vi "main_1 displacement detection.vi"() -> ()   [LabVIEW 2024]
doc: "This example shows how to configure multiple channels and acquire waveforms from multiple channels."
uses:
  RIGOL DS5000 7000 8000 Series/Public/Data/Read Waveform (Multiple).vi
  <vilib>/measure/mamon.llb/Waveform Peak Detection for 1 Chan.vi
  <vilib>/express/express analysis/Spectral/Block/exnSpectralBlock spectral measurements peak poly.vi
  <vilib>/express/express analysis/Spectral/Block/exnSpectralBlock spectral measurements peak WFM.vi
  <vilib>/Utility/file.llb/Write Delimited Spreadsheet (string).vi
  <vilib>/express/express analysis/Spectral/XNode/ExpressSpectralMeasurementsBlockNode.xnode
  RIGOL DS5000 7000 8000 Series/RIGOL DS5000 7000 8000 Series.lvlib
  <vilib>/measure/NI_MAPro.lvlib
panel:
  in  "Reset":bool
  in  "Negative direction":bool
  out "位移":dbl(graph)
  out "字符串":string
  in  "确定按钮":bool
  out "布尔 2":bool
  in  "Threshold":dbl=0.15
  in  "Save":bool
  out "Frequency":dbl
  in  "Time":dbl=20.0
  out "下拉列表":u16(ring)
  out "Count":dbl
  out "0, 1":i16
  out "子数组":dbl[](array[numeric])
  out "大小":i32
  out "# found":i32 caption="Count"
  in  "记时长度":dbl format="%#_13g"
  in  "Threshold":dbl=1.0
  out "Real time FFT":cluster{"f0":dbl, "df":dbl, "magnitude":dbl[]}(graph)
  out "输出数组":string[][](array[string])
  in  "停止":bool
  in  "Data format":string=".xls"
  in  "连接":bool
  in  "Data saving path":path
  in  "选项卡控件":enum32{"Channel 1", "Channel 2"}(tab)
  in  "Channel Number":u16(ring)=1 items=["Channel 1"=1, "Channel 2"=2]
  in  "电流方式":u16(ring)=1 items=["AC", "DC", "Ground"]
  in  "Probe Attenuation":u16(ring)=6 items=["0.01X", "0.02X", "0.05X", "0.1X", "0.2X", "0.5X", "1X", "2X", "5X", "10X", "20X", "50X", "100X", "200X", "500X", "1000X", "2000X", "5000X", "10000X", "20000X", "50000X"]
  in  "Time per Division (0.0005 s)":dbl=1e-07
  in  "Record Length (10k points)":u32=100000
  in  "Channel (2: Channel 2)":u16(ring)=2 items=["Channel 1"=1, "Channel 2"=2]
  in  "Vertical Coupling (1: DC)":u16(ring)=1 items=["AC", "DC", "Ground"]
  in  "Probe Attenuation  2":u16(ring)=6 items=["0.01X", "0.02X", "0.05X", "0.1X", "0.2X", "0.5X", "1X", "2X", "5X", "10X", "20X", "50X", "100X", "200X", "500X", "1000X", "2000X", "5000X", "10000X", "20000X", "50000X"]
  out "Received signal":waveform(dbl)[](graph)
  in  "Serial port":refnum<visa-resource-name>
  # "Chip-less Wireless Sensing System"
  # "Control panel"
  # "Count"
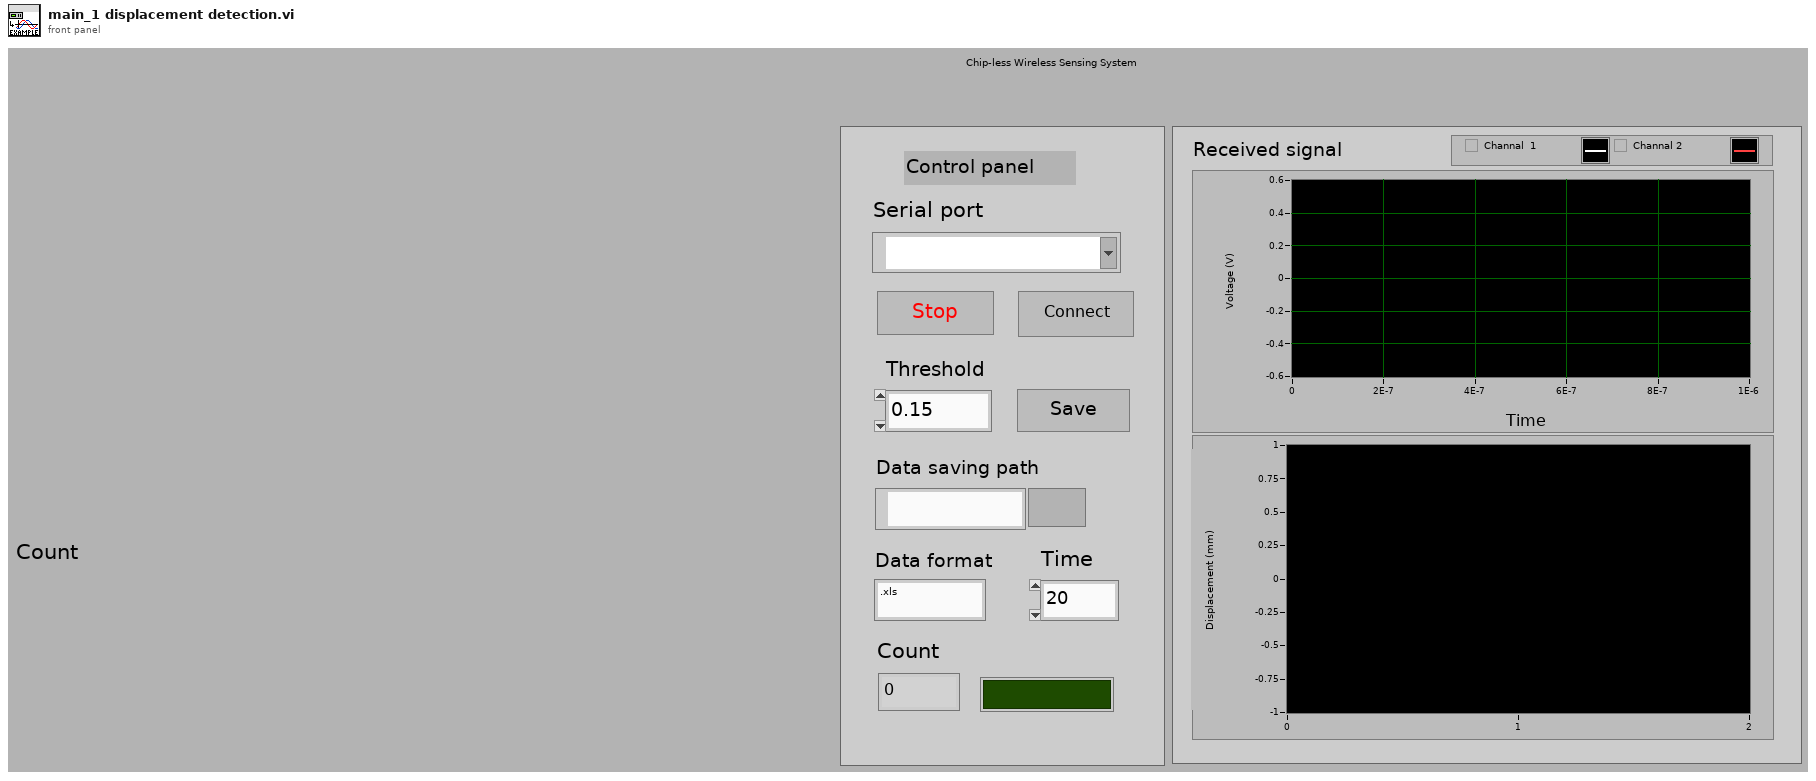
[diagram p1: front panel]
types:
  T1 = cluster{"averaging mode":u16, "weighting mode":u16, "number of averages":u32}
  T2 = cluster{"dB On (F)":bool, "unwrap phase (F)":bool, "convert to degree (F)":bool}
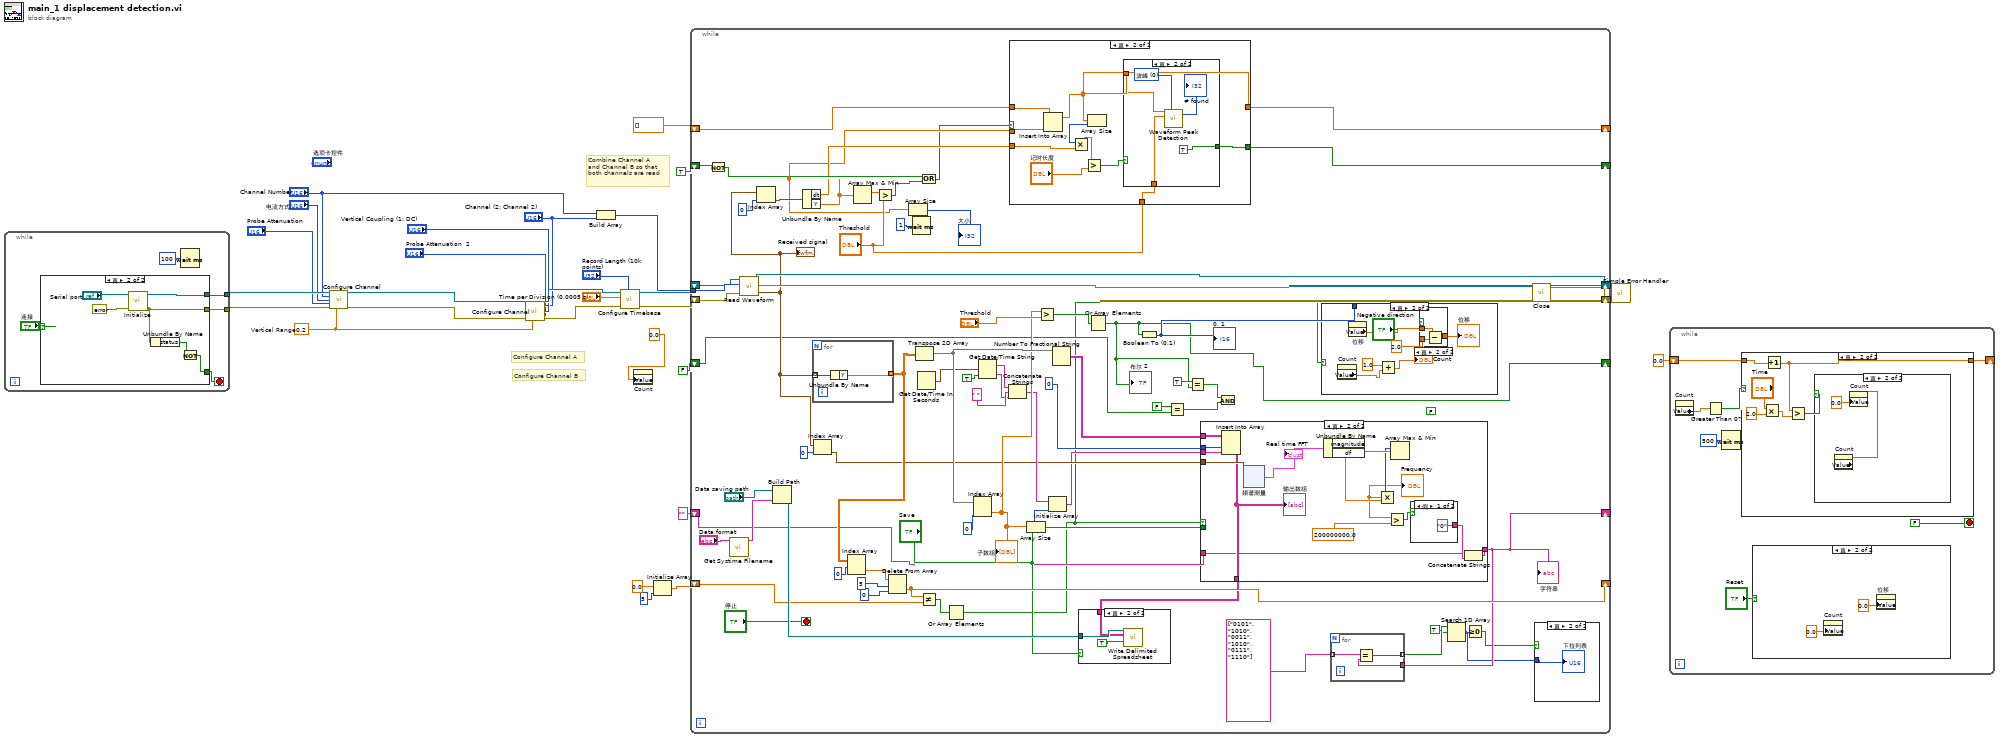
[diagram p0: block diagram]
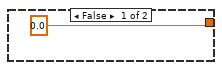
[diagram p3: hidden frame]
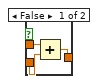
[diagram p7: hidden frame]
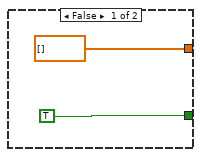
[diagram p8: hidden frame]
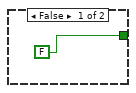
[diagram p9: hidden frame]
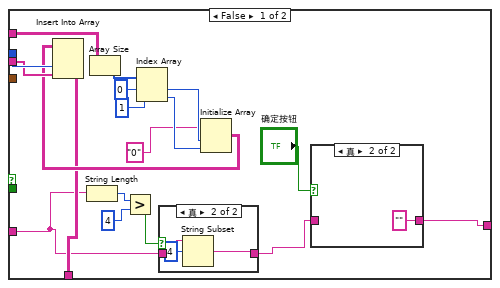
[diagram p11: hidden frame]
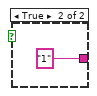
[diagram p14: hidden frame]
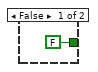
[diagram p15: hidden frame]
diagram:
  w23 = 0.2  # Vertical Range
  # "Combine Channel A\nand Channel B so that\nboth channels are read"
  # "Configure Channel B"
  # "Configure Channel A"
  n1 = while {
    tunnel: [w35] -> w29
    tunnel: [w34] -> w28
    stop <- w33 stop-if-true
    n2 = case shown="真" "连接" {
      tunnel: [_ w41] -> w35
      tunnel: [_ w39] -> w34
      tunnel: [FALSE w37] -> w33
      frame False {
      }
      frame True {
        n3 = call "Initialize.vi"("error in (no error)"=errorcluster {"status"=FALSE, "code"=0, "source"=""}, "VISA resource name"="Serial port") -> ("error out"=w39:errorcluster, "VISA resource name out"=w41:refnum<visa-resource-name>)  [unwired: 8 in]
        n4 = Unbundle By Name(w39) -> ("status"=w38:bool)
        n5 = Not(x=w38) -> (.not. x?=w37:bool)
      }
    }
    n6 = Wait (ms)(milliseconds to wait=u32 100 ("等待时间（毫秒）")) -> ()  [unwired: 1 out]
  }
  n7 = call "Configure Channel.vi"("VISA resource name"=w29, "Channel (1: Channel 1)"="Channel Number", "Vertical Coupling (1: DC)"="电流方式", "Probe Attenuation"="Probe Attenuation", "error in (no error)"=w28, "Vertical Range (10.0 V)"=w23) -> ("VISA resource name out"=w20:refnum<visa-resource-name>, "error out"=w19:errorcluster)  [unwired: 8 in]
  n8 = call "Configure Channel.vi"("VISA resource name"=w20, "Channel (1: Channel 1)"="Channel (2: Channel 2)", "Vertical Coupling (1: DC)"="Vertical Coupling (1: DC)", "Probe Attenuation"="Probe Attenuation  2", "error in (no error)"=w19, "Vertical Range (10.0 V)"=w23) -> ("VISA resource name out"=w27:refnum<visa-resource-name>, "error out"=w26:errorcluster)  [unwired: 8 in]
  n9 = Build Array("Channel Number", "Channel (2: Channel 2)") -> (w15:u16[])
  n10 = call "Configure Timebase.vi"("Record Length (10k points)"="Record Length (10k points)", "error in (no error)"=w26, "Time per Division (0.0005 s)"="Time per Division (0.0005 s)", "VISA resource name"=w27) -> ("error out"=w16:errorcluster, "VISA resource name out"=w14:refnum<visa-resource-name>)  [unwired: 6 in]
  n11 = property on="Count" class="DigNum (严格)"("Value"=0.0) -> ()  [unwired: 2 in, 2 out]
  n12 = Initialize Array(0.0, 5 ("维数大小")) -> (w7:dbl[])
  n13 = while {
    tunnel: w15 -> [w107]
    shift-right: [w109] -> w17
    shift-left: w16 -> [w108]
    shift-right: [w110] -> w18
    shift-left: w14 -> [w106]
    shift-right: [w82] -> _
    shift-left: w7 -> [w83]
    shift-right: [w66] -> _
    shift-left: dbl[] [] -> [w67]
    shift-right: [w64] -> _
    shift-left: TRUE -> [w69]
    shift-right: [w52] -> _
    shift-left: FALSE -> [w58]
    shift-right: [w50] -> _
    shift-left: "" -> [w45]
    stop <- "停止" stop-if-true
    (unwired) FALSE
    n14 = Not(x=w69) -> (.not. x?=w68:bool)
    n15 = call "Get Systime Filename.vi"("文件格式"="Data format") -> ("输出时间文件"=w103:string)  [unwired: 10 in]
    n16 = call-poly "Read Waveform.vi"("error in (no error)"=w108, "Channels"=w107, "VISA resource name"=w106) -> ("error out"=w109:errorcluster, "Waveform Data"=w74:waveform(dbl)[], "VISA resource name out"=w110:refnum<visa-resource-name>)  [unwired: 6 in]
    "Received signal" <- w74
    n17 = Index Array(array=w74, index=0 ("索引")) -> (element=w72:waveform(dbl))
    n18 = Build Path(base path="Data saving path", name or relative path=w103) -> (appended path=w102:path)
    n19 = Unbundle By Name(w72) -> ("dt"=w65:dbl, "Y"=w62:dbl[])
    n20 = for {
      tunnel: w74 -> [w201] mode=indexing
      tunnel: [w200] -> w88 mode=indexing
      n21 = Unbundle By Name(w201) -> ("Y"=w200:dbl[])
    }
    n22 = Index Array(array=w74, index=0 ("索引 (行)")) -> (element=w79:waveform(dbl))
    n23 = Index Array(array=w88, index (row)=0 ("索引 (行)")) -> (element=w86:dbl[])  [unwired: 1 in]
    n24 = Array Max & Min(array=w62) -> (max value=w71:dbl)  [unwired: 3 out]
    n25 = Greater?(x=w71, y="Threshold") -> (0:w70:bool)
    n26 = Delete From Array(array=w86, length=5 ("长度"), index=0 ("索引")) -> (deleted portion=w82:dbl[])  [unwired: 1 out]
    n27 = Array Size(array=w62) -> (size(s)=→"大小":i32)
    n28 = Wait (ms)(milliseconds to wait=u32 1 ("等待时间（毫秒）")) -> ()  [unwired: 1 out]
    n29 = Transpose 2D Array(2D array=w88) -> (transposed array=w100:dbl[][])
    n30 = Get Date/Time In Seconds() -> (seconds since 1Jan1904=w89:timestamp)
    n31 = Or(x=w68, y=w70) -> (x .or. y?=w44:bool)
    n32 = Not Equal?(x=w82, y=w83) -> (x != y?=w81:bool[])
    n33 = Or Array Elements(Boolean array=w81) -> (logical OR=w43:bool)
    n34 = Index Array(array=w100, index (col)=0 ("禁用的索引 (列)")) -> (element=w93:dbl[])  [unwired: 1 in]
    "子数组" <- w93
    n35 = Get Date/Time String(seconds (now)=w89, want seconds? (F)=TRUE ("需要秒？(F)")) -> (date string=w95:string, time string=w96:string)  [unwired: 1 in]
    n36 = Concatenate Strings(w95, " " ("字符串"), w96) -> (w92:string)
    n37 = case shown="真" w44 {
      tunnel: w62 -> [_ w139]
      tunnel: w67 -> [_ w138]
      tunnel: [dbl[] [] w131] -> w66
      tunnel: w65 -> [_ w136]
      tunnel: [TRUE w132] -> w64
      tunnel: "Threshold" -> [_ w130]
      frame False {
      }
      frame True {
        n38 = Insert Into Array(array=w138, new element=w139) -> (w131:dbl[])  [unwired: 1 in]
        n39 = Array Size(array=w131) -> (size(s)=w137:i32)
        n40 = Multiply(x=w137, y=w136) -> (x*y=w135:dbl)
        n41 = Greater?(x=w135, y="记时长度") -> (0:w133:bool)
        n42 = case shown="真" w133 {
          tunnel: [FALSE TRUE] -> w132
          tunnel: w131 -> [_ w144]
          tunnel: w130 -> [_ w143]
          frame False {
          }
          frame True {
            w142 = u16 0 items=["波峰", "波谷"] ("peaks/valleys")
            n43 = call-poly <vilib>:"Waveform Peak Detection.vi"("peaks/valleys"=w142, "threshold"=w143, "Signal In"=w144) -> ("# found"=→"# found":i32)  [unwired: 4 in, 4 out]
          }
        }
      }
    }
    n44 = Array Size(array=w93) -> (size(s)=w91:i32)
    n45 = Greater?(x=w93, y="Threshold") -> (0:w60:bool[])
    n46 = Initialize Array(w92, w91) -> (w75:string[])
    n47 = Number To Fractional String(number=w100) -> (F-format string=w77:string[][])  [unwired: 3 in]
    n48 = Or Array Elements(Boolean array=w60) -> (logical OR=w52:bool)
    "布尔 2" <- w52
    n49 = Boolean To (0,1)(Boolean=w52) -> (0, 1=w59:i16)
    "0, 1" <- w59
    n50 = Equal?(x=FALSE, y=w58) -> (x = y?=w54:bool)
    n51 = Equal?(x=TRUE, y=w52) -> (x = y?=w55:bool)
    n52 = case shown="真" w43 {
      tunnel: "Save" -> [_ _]
      tunnel: w79 -> [_ w187]
      tunnel: [w156 w183] -> w78
      tunnel: w77 -> [w158 w186]
      tunnel: 0 ("禁用的索引 (列)") -> [w160 w184]
      tunnel: w75 -> [w159 w185]
      tunnel: [w155 w174] -> w50
      tunnel: w45 -> [w150 w173]
      frame False {
        n53 = String Length(string=w150) -> (length=w153:i32)
        n54 = Array Size(array=w158) -> (size(s)=w166:i32[])
        n55 = Greater?(x=w153, y=4) -> (0:w151:bool)
        n56 = Index Array(array=w166, index #1=0 ("索引"), index #2=1 ("索引")) -> (element #1=w163:i32, element #2=w162:i32)
        n57 = case shown="真" w151 {
          tunnel: w150 -> [w167 w170]
          tunnel: [w167 w168] -> w149
          frame False {
          }
          frame True {
            n58 = String Subset(string=w170, offset (0)=4 ("偏移量(0)")) -> (substring=w168:string)  [unwired: 1 in]
          }
        }
        n59 = Initialize Array("0", w163, w162) -> (w157:string[][])
        n60 = Insert Into Array(array=w157, index (col)=w160, new element=w159) -> (w156:string[][])  [unwired: 1 in]
        n61 = case shown="真" "确定按钮" {
          tunnel: w149 -> [w171 _]
          tunnel: [w171 ""] -> w155
          frame False {
          }
          frame True {
          }
        }
      }
      frame True {
        n62 = Insert Into Array(array=w186, index (col)=w184, new element=w185) -> (w183:string[][])  [unwired: 1 in]
        "输出数组" <- w183
        n63 = xnode "频谱测量"("信号"=w187) -> ("FFT - （峰值）"=w182:cluster{"f0":dbl, "df":dbl, "magnitude":dbl[]})  [unwired: 1 in, 2 out]
        "Real time FFT" <- w182
        n64 = Unbundle By Name(w182) -> ("magnitude"=w181:dbl[], "df"=w179:dbl)
        n65 = Array Max & Min(array=w181) -> (max index (indices)=w180:i32)  [unwired: 3 out]
        n66 = Multiply(x=w180, y=w179) -> (x*y=w178:dbl)
        "Frequency" <- w178
        n67 = Greater?(x=w178, y=200000000.0) -> (0:w176:bool)
        n68 = case shown="假" w176 {
          tunnel: ["0" "1"] -> w175
          frame False {
          }
          frame True {
          }
        }
        n69 = Concatenate Strings(w173, w175) -> (w174:string)
      }
    }
    "字符串" <- w50
    n70 = case shown="真" "Save" {
      tunnel: w102 -> [_ w148]
      tunnel: w78 -> [_ w146]
      frame False {
      }
      frame True {
        n71 = call-poly <vilib>:"Write Delimited Spreadsheet.vi"("file path (dialog if empty)"=w148, "2D data"=w146, "append to file? (new file:F)"=TRUE) -> ()  [unwired: 11 in, 2 out]
      }
    }
    n72 = And(x=w55, y=w54) -> ()  [unwired: 1 out]
    n73 = case shown="真" w43 {
      tunnel: w59 -> [_ _]
      frame False {
      }
      frame True {
        n74 = property on="Count" class="DigNum (严格)"() -> ("Value"=w121:dbl)  [unwired: 2 in, 2 out]
        n75 = property on="位移" class="WFChart (严格)"() -> ("Value"=w117:dbl)  [unwired: 2 in, 2 out]
        n76 = Add(x=1.0, y=w121) -> (x+y=→"Count":dbl)
        n77 = case shown="真" "Negative direction" {
          tunnel: 2.0 ("y") -> [w124 w127]
          tunnel: w117 -> [w123 w125]
          tunnel: [w122 w126] -> w116
          frame False {
            n78 = Add(x=w123, y=w124) -> (x+y=w122:dbl)
          }
          frame True {
            n79 = Subtract(x=w125, y=w127) -> (x-y=w126:dbl)
          }
        }
        "位移" <- w116
      }
    }
    n80 = for {
      tunnel: string[] ["0101", "1010", "0011", "1010", "0111", "1110"] -> [w114] mode=indexing
      tunnel: w50 -> [w113]
      tunnel: [w112] -> w49 mode=indexing
      n81 = Equal?(x=w114, y=w113) -> (x = y?=w112:bool)
    }
    n82 = Search 1D Array(1D array=w49, element=TRUE ("元素")) -> (index of element=w46:i32)  [unwired: 1 in]
    n83 = Greater Or Equal To 0?(x=w46) -> (x >= 0?=w47:bool)
    n84 = case shown="真" w47 {
      tunnel: w46 -> [_ w111]
      frame False {
      }
      frame True {
        "下拉列表" <- w111
      }
    }
  }
  n85 = call "Close.vi"("error in (no error)"=w17, "VISA resource name"=w18) -> ("error out"=w30:errorcluster)  [unwired: 9 in]
  n86 = call <vilib>:"Simple Error Handler.vi"("error in (no error)"=w30) -> ()  [unwired: 4 in, 5 out]
  n87 = while {
    shift-right: [w204] -> _
    shift-left: 0.0 -> [w205]
    stop <- FALSE stop-if-true
    n88 = property on="Count" class="DigNum (严格)"() -> ("Value"=w207:dbl)  [unwired: 2 in, 2 out]
    n89 = Greater Than 0?(x=w207) -> (x > 0?=w206:bool)
    n90 = Wait (ms)(milliseconds to wait=u32 500 ("等待时间（毫秒）")) -> ()  [unwired: 1 out]
    n91 = case shown="真" w206 {
      tunnel: w205 -> [_ w217]
      tunnel: [0.0 w216] -> w204
      frame False {
      }
      frame True {
        n92 = Multiply(x="Time", y=2.0) -> (x*y=w215:dbl)
        n93 = Increment(x=w217) -> (x+1=w216:dbl)
        n94 = Greater?(x=w216, y=w215) -> (0:w212:bool)
        n95 = case shown="真" w212 {
          frame False {
          }
          frame True {
            n96 = property on="Count" class="DigNum (严格)" props=["Value"]() -> (error out=w218:errorcluster)  [unwired: 2 in, 2 out]
            n97 = property on="Count" class="DigNum (严格)"(error in=w218, "Value"=0.0 ("震荡计数")) -> ()  [unwired: 1 in, 2 out]
          }
        }
      }
    }
    n98 = case shown="真" "Reset" {
      frame False {
      }
      frame True {
        n99 = property on="Count" class="DigNum (严格)"("Value"=0.0 ("Count")) -> ()  [unwired: 2 in, 2 out]
        n100 = property on="位移" class="WFChart (严格)"("Value"=0.0 ("位移")) -> ()  [unwired: 2 in, 2 out]
      }
    }
  }
